vi "PixyCam_Close.vi"(4 "error in":errorcluster, 7 "PixyCamDevRef":T1) -> (0 "error out":errorcluster)   [LabVIEW 2016, in "PixyCam_LabVIEW.lvlib"]
uses:
  PixyCam_LabVIEW.lvlib
  Private/PixyCam_DevRef.ctl
  Private/PixyCam_SPI_DevRef.ctl
  <vilib>/Rock Robotics/WPI/SPI/WPI_SPIDevRef.ctl
  <vilib>/Rock Robotics/SystemInterfaces/spilib/spi_bus.ctl
  Private/PixyCam_CommMode.ctl
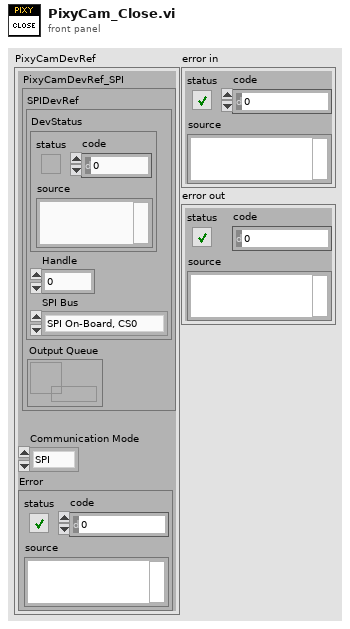
[diagram p1: front panel]
types:
  T1 = typedef "PixyCam_LabVIEW.lvlib/PixyCam_DevRef.ctl" = cluster{"PixyCamDevRef_SPI":T2, "Communication Mode":T5, "Error":errorcluster}
  T2 = typedef "PixyCam_LabVIEW.lvlib/PixyCam_SPI_DevRef.ctl" = cluster{"SPIDevRef":T3, "Output Queue":refnum<queue>}
  T3 = typedef "WPI_SPIDevRef.ctl" = cluster{"DevStatus":errorcluster, "Handle":i32, "SPI Bus":T4}
  T4 = typedef "spi_bus.ctl" = enum16{"SPI On-Board, CS0", "SPI On-Board, CS1", "SPI On-Board, CS2", "SPI On-Board, CS3", "SPI MXP", "Invalid"}
  T5 = typedef "PixyCam_LabVIEW.lvlib/PixyCam_CommMode.ctl" = enum16{"SPI", "I2C", "UART", "Analog", "Digital"}
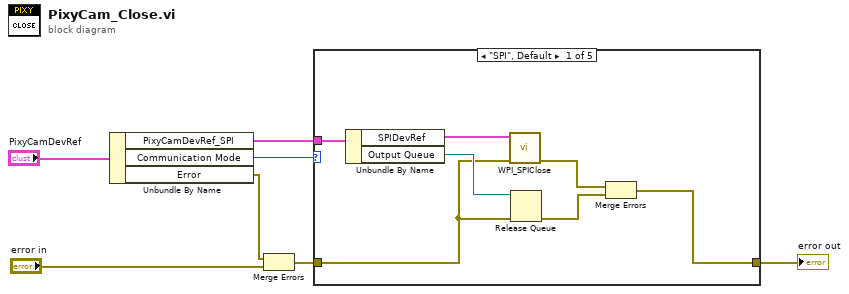
[diagram p0: block diagram]
diagram:
  n1 = Unbundle By Name("PixyCamDevRef") -> ("PixyCamDevRef_SPI"=w5:T2, "Communication Mode"=w6:T5, "Error"=w4:errorcluster)
  n2 = Merge Errors(w4, "error in") -> (w2:errorcluster)
  n3 = case shown="\"SPI\", Default" w6 {
    tunnel: w5 -> [w14 _ _ _ _]
    tunnel: w2 -> [w11 w15 w16 w17 w18]
    tunnel: [w8 w15 w16 w17 w18] -> w1
    frame "SPI", Default {
      n4 = Unbundle By Name(w14) -> ("SPIDevRef"=w12:T3, "Output Queue"=w13:refnum<queue>)
      n5 = call <vilib>:"WPI_SPIClose.vi"("error in (no error)"=w11, "SPIDevRef"=w12) -> ("error out"=w10:errorcluster)  [unwired: 9 in]
      n6 = Release Queue(queue=w13, error in (no error)=w11) -> (error out=w9:errorcluster)  [unwired: 1 in, 2 out]
      n7 = Merge Errors(w10, w9) -> (w8:errorcluster)
    }
    frame "I2C" {
    }
    frame "UART" {
    }
    frame "Analog" {
    }
    frame "Digital" {
    }
  }
  "error out" <- w1
